vi "Walsh Hadamard Inverse.vi"(0 "X":dbl[](array[numeric])) -> (1 "Walsh Hadamard Inverse {X}":dbl[](array[numeric]), 2 "error":i32)   [LabVIEW 2018, in "NI_Gmath.lvlib"]
doc: "Computes the inverse of the real Walsh Hadamard transform of the input sequence <B>X</B>."
uses:
  NI_Gmath.lvlib
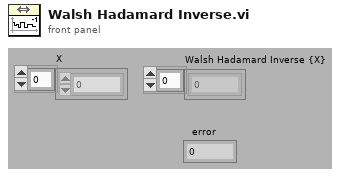
[diagram p1: front panel]
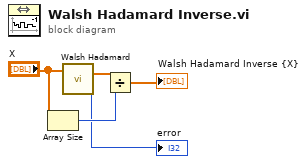
[diagram p0: block diagram]
diagram:
  n1 = Array Size(array="X") -> (size(s)=w3:i32)
  n2 = call "Walsh Hadamard.vi"("X"="X") -> ("Walsh Hadamard {X}"=w5:dbl[], "error"=→"error":i32)
  n3 = Divide(x=w5, y=w3) -> (x/y=→"Walsh Hadamard Inverse {X}":dbl[])
